vi "Get DAT Name.vi"(8 "error in (no error)":errorcluster caption="错误输入（无错误）", 11 "Waveform":waveform(dbl) caption="波形") -> (0 "error out":errorcluster caption="错误输出", 1 "File Name":string caption="文件名", 3 "File Path":path caption="文件路径")   [LabVIEW 2013]
uses:
  Globals/Global - Configuration Options.vi
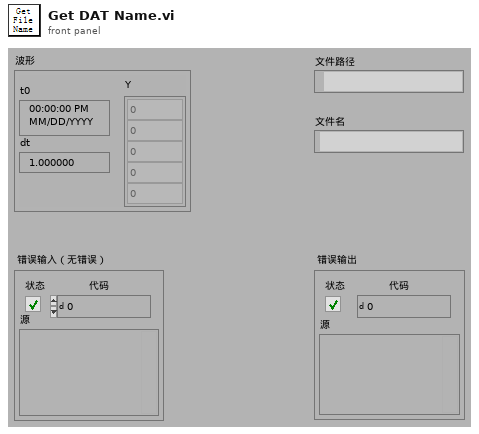
[diagram p1: front panel]
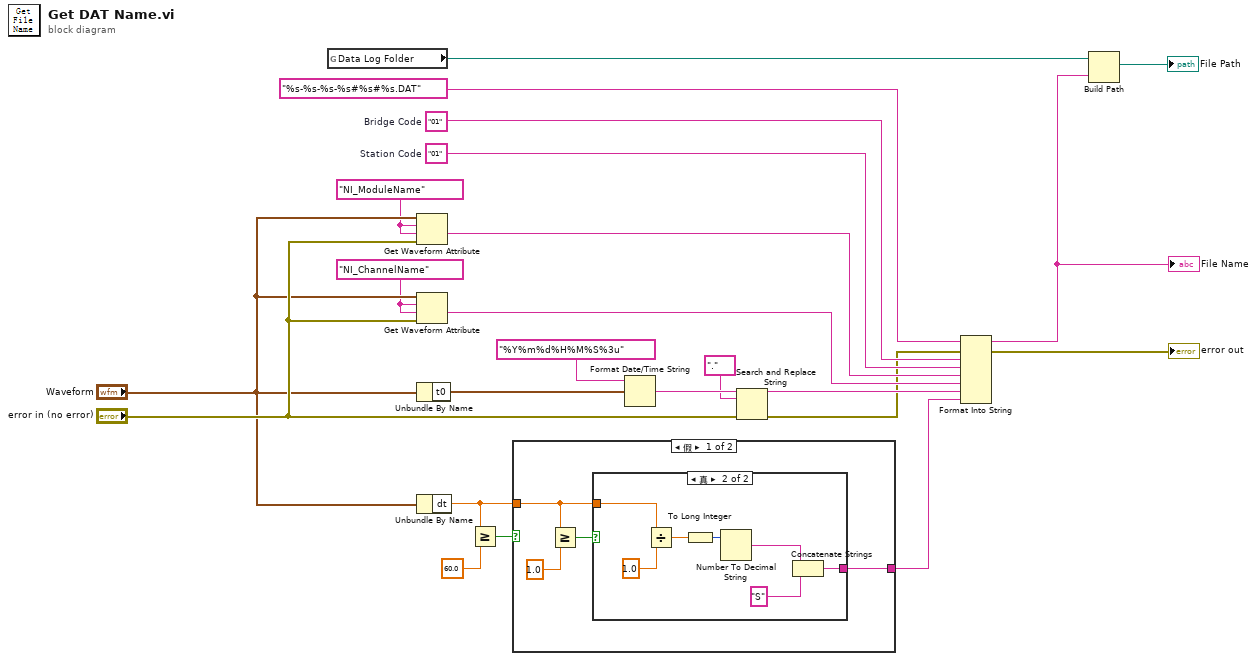
[diagram p0: block diagram]
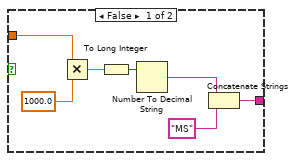
[diagram p2: hidden frame]
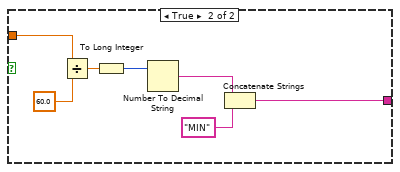
[diagram p3: hidden frame]
diagram:
  w1 = "NI_ChannelName" ("名称")
  w2 = "NI_ModuleName" ("名称")
  w20 = "01"  # Station Code
  w21 = "01"  # Bridge Code
  n1 = global read "Global - Configuration Options.vi" "Data Log Folder"() -> (w10:path)
  n2 = Get Waveform Attribute(4:"error in (no error)", 5:w2, 6:w2, 7:"Waveform") -> (1:w8:string)  [unwired: 3 out]
  n3 = Get Waveform Attribute(4:"error in (no error)", 5:w1, 6:w1, 7:"Waveform") -> (1:w7:string)  [unwired: 3 out]
  n4 = Unbundle By Name("Waveform") -> ("t0"=w9:timestamp)
  n5 = Unbundle By Name("Waveform") -> ("dt"=w5:dbl)
  n6 = Greater Or Equal?(x=w5, y=60.0) -> (x >= y?=w17:bool)
  n7 = case shown="假" w17 {
    tunnel: w5 -> [w25 w48]
    tunnel: [w24 w42] -> w14
    frame False {
      n8 = Greater Or Equal?(x=w25, y=1.0) -> (x >= y?=w26:bool)
      n9 = case shown="真" w26 {
        tunnel: w25 -> [w29 w36]
        tunnel: [w28 w35] -> w24
        frame False {
          n10 = Multiply(x=w29, y=1000.0) -> (x*y=w33:dbl)
          n11 = To Long Integer(number=w33) -> (32bit integer=w32:i32)
          n12 = Number To Decimal String(number=w32) -> (decimal integer string=w31:string)  [unwired: 1 in]
          n13 = Concatenate Strings(w31, "MS" ("字符串")) -> (w28:string)
        }
        frame True {
          n14 = Divide(x=w36, y=1.0) -> (x/y=w40:dbl)
          n15 = To Long Integer(number=w40) -> (32bit integer=w39:i32)
          n16 = Number To Decimal String(number=w39) -> (decimal integer string=w38:string)  [unwired: 1 in]
          n17 = Concatenate Strings(w38, "S" ("字符串")) -> (w35:string)
        }
      }
    }
    frame True {
      n18 = Divide(x=w48, y=60.0) -> (x/y=w46:dbl)
      n19 = To Long Integer(number=w46) -> (32bit integer=w45:i32)
      n20 = Number To Decimal String(number=w45) -> (decimal integer string=w44:string)  [unwired: 1 in]
      n21 = Concatenate Strings(w44, "MIN" ("字符串")) -> (w42:string)
    }
  }
  n22 = Format Date/Time String(time format string (%c)="%Y%m%d%H%M%S%3u" ("时间格式字符串(%c)"), seconds (now)=w9) -> (date/time string=w13:string)  [unwired: 1 in]
  n23 = Search and Replace String(input string=w13, search string="." ("搜索字符串"), error in="error in (no error)") -> (result string=w12:string, error out=w6:errorcluster)  [unwired: 5 in, 2 out]
  n24 = Format Into String(format string="%s-%s-%s-%s#%s#%s.DAT" ("格式字符串"), error in=w6, w21, w20, w8, w7, w12, w14) -> (resulting string=w19:string, error out=→"error out":errorcluster)  [unwired: 1 in]
  "File Name" <- w19
  n25 = Build Path(base path=w10, name or relative path=w19) -> (appended path=→"File Path":path)
